vi "sub.vi"() -> ()   [LabVIEW 2026]
panel:
  out "output":dbl
  in  "b":dbl
  in  "a":dbl
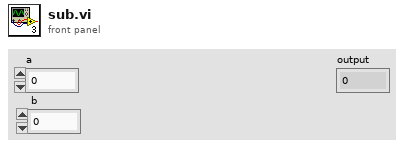
[diagram p1: front panel]
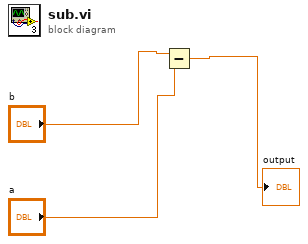
[diagram p0: block diagram]
diagram:
  n1 = Subtract(x="b", y="a") -> (x-y=→"output":dbl)
